vi "Dashboard_Main_Fixed_1366_768.vi"() -> ()   [LabVIEW 2023]
uses:
  <vilib>/event_ctls.llb/eventvkey.ctl
  <vilib>/Rock Robotics/Network Tables/NT Read Numeric Array.vi
  <vilib>/Rock Robotics/WPI/Dashboard/WPI_DashboardLogging Global.vi
panel:
  in  "Camera Settings Right":T1={"Frame Rate"=30, "Compression"=30, "Size"=1, "DB Camera Config"=FALSE} {"Frame Rate" scale=1.0..30.0; "Compression" scale=100.0..-1.0; "Size" items=["640x480", "320x240", "160x120"]}
  in  "Camera Name Right":string(combo)="No Camera Selection"
  out "Camera Perf":string
  in  "Camera Settings":T1={"Frame Rate"=30, "Compression"=30, "Size"=1, "DB Camera Config"=FALSE} {"Frame Rate" scale=1.0..30.0; "Compression" scale=100.0..-1.0; "Size" items=["640x480", "320x240", "160x120"]}
  in  "TCP":refnum<k5>
  in  "Rec Mode":enum32{"Stop", "Record", "Playback"}(radio)
  out "Robot IP":string
  out "Image Message":string="Timeout in Camera Communications"
  in  "Dashboard Tab":T2(tab)
  in  "Select Auto":string(combo)="Select Autonomous ..."
  out "NT Connection":bool
  out "MotorChart R":cluster{"Numeric":dbl, "Numeric":dbl}(graph)
  out "MotorChart L":cluster{"Numeric":dbl, "Numeric":dbl}(graph)
  out "MotorSliders R":cluster{"MotorSlide1":dbl, "MotorSlide2":dbl} {"MotorSlide2" scale=-1.0..1.0 scale format="%#_2e"; "MotorSlide1" scale=-1.0..1.0 scale format="%#_2e"}
  out "MotorSliders L":cluster{"MotorSlide1":dbl, "MotorSlide2":dbl} {"MotorSlide2" scale=-1.0..1.0 scale format="%#_2e"; "MotorSlide1" scale=-1.0..1.0 scale format="%#_2e"}
  out "Gyro":dbl(knob) scale=0.0..360.0
  out "JS1 Z":dbl(slide) scale=-1.0..1.0 scale format="%#_2e"
  out "JS1 Graph":cluster{"X":dbl, "Y":dbl}[](graph)
  out "JS1 Buttons":T3
  out "JS2 Z":dbl(slide) scale=-1.0..1.0 scale format="%#_2e"
  out "JS2 Graph":cluster{"X":dbl, "Y":dbl}[](graph)
  out "JS2 Buttons":T3
  out "Mode":T4(ring)=enum."Auto Disabled"
  out "Right Camera Perf":cluster{"Bandwidth (Mbps)":dbl, "FPS":dbl}
  out "Camera Image Right":T5(plugin-control)
  in  "DB/String 9":string
  in  "DB/String 8":string
  in  "DB/String 7":string
  in  "DB/String 6":string
  in  "DB/String 5":string
  in  "DB/String 4":string
  in  "DB/String 3":string
  in  "DB/String 2":string
  in  "DB/String 1":string
  in  "DB/String 0":string
  in  "DB/Slider 0":dbl(slide) scale=0.0..5.0
  in  "DB/Slider 1":dbl(slide) scale=0.0..5.0
  in  "DB/Slider 2":dbl(slide) scale=0.0..5.0
  in  "DB/Slider 3":dbl(slide) scale=0.0..5.0
  out "DB/LED 3":bool
  out "DB/LED 2":bool
  out "DB/LED 1":bool
  out "DB/LED 0":bool
  in  "DB/Button 3":bool
  in  "DB/Button 2":bool
  in  "DB/Button 1":bool
  in  "DB/Button 0":bool caption="New Name"
  in  "Test Slider":dbl(slide) scale=0.0..100.0 scale format="%#_3g"
  in  "On/Off":bool caption="Solenoid"
  in  "Test Name":u16(ring) items=["Select the test to run..."]
  in  "Test Tree":string(tree)
  in  "Motor":cluster{"Value":dbl, "Enable":bool} {"Value" scale=-1.0..1.0 scale format="%#_3g"}
  out "Progress":T6 {"Test Progress" scale=0.0..100.0}
  in  "Rev/Fwd":cluster{"Forward":bool, "Reverse":bool}
  in  "Test Ring":u16(ring) items=["Monochrome", "Color"]
  in  "CheckList":i32(listbox)
  out "Tree":string(tree)
  out "Camera Image":T5(plugin-control)
  out "Background":bool
  in  "Camera Name":string(combo)="No Camera Selection"
  # "HW"
  # "HW"
  # "Joysticks"
  # "Drive Motors"
  # "Front"
  # "Right"
  # "Left"
  # "Back"
  # "This tab is a great place for autonomous settings and robot-specific values.\nPlace controls and indicators inside this tab and match name to\nDashboard Variables on robot. You can also delete this comment."
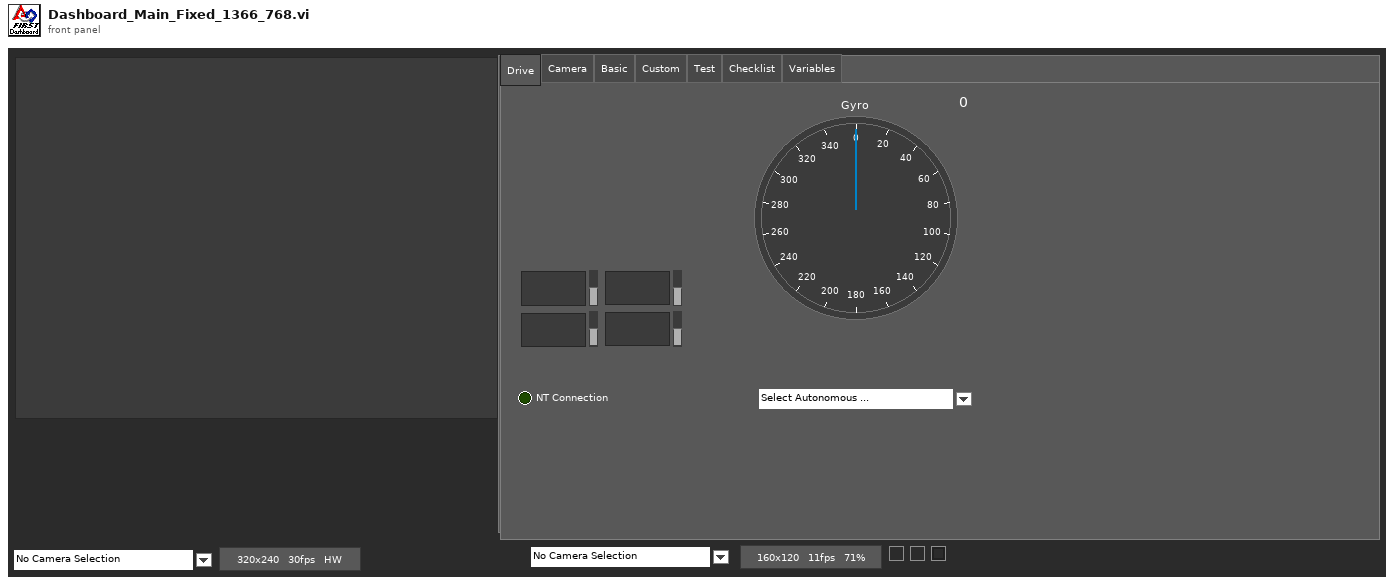
[diagram p1: front panel]
types:
  T1 = cluster{"Frame Rate":i32, "Compression":i32, "Size":u16, "DB Camera Config":bool}
  T2 = enum32{"Drive", "Camera", "Basic", "Custom", "Test", "Checklist", "Variables"}
  T3 = cluster{bool, bool, bool, bool, bool, bool, bool, bool, bool, bool, bool, bool}
  T4 = enum8{"Tele-Op Disabled", "Tele-Op Enabled", "Auto Disabled", "Auto Enabled", "Test Disabled", "Test Enabled", "Disconnected", "No Code", "E-Stop"}
  T5 = typedef "IMAQ Image.ctl" = refnum<image>
  T6 = cluster{"Test Progress":u8, "Test Progress Text":string}
  T7 = cluster{"Save Path":path, "Interval (s)":dbl, "Keep":i32}
  T8 = enum32{"Drive", "Camera", "Basic", "Custom", "Test", "Commands", "Checklist", "Variables"}
  T9 = typedef "Image Type" = u32
  T10 = cluster{"Error Strings":string, "Disable Counts":cluster{u16, u16}, "Rail Faults":cluster{u16, u16, u16}, "Robot IP":string, "DB Mode":u8, "Event Info":cluster{"Name":string, "Type":u8, "Number":u16, "Replay":u8}}
  T11 = cluster{"Storage":cluster{"Disk Free":u64, "RAM Block":u32, "RAM free":u32}, "CPU Utilization":cluster{"CPU % ISR":sgl, "CPU % Time Crit":sgl, "CPU % Timed Str":sgl, "CPU % High":sgl, "CPU % Above":sgl, "CPU % Normal":sgl, "CPU % Low":sgl}, "CAN":cluster{"% Bus Utilization":sgl, "Bus Off Cnt":u32, "TX_FIFO Full Cnt":u32, "Receive Error Cnt":u8, "Transmit Error Cnt":u8}, "HID":cluster{"HID Outputs":u32, "Rumble Low":u16, "Rumble High":u16}[]}
  T12 = cluster{"Status bits":cluster{"Test Mode":bool, "Autonomous":bool, "Enabled":bool, "Code Start":bool, "Brownout":bool, "Reserved 2":bool, "Reserved 3":bool, "E-Stop":bool}, "Code Trace":cluster{"Disabled":bool, "TeleOp":bool, "Auto":bool, "Test":bool}, "Controller Type":enum16{"unknown", "cRIO", "roboRio"}, "Code?":enum16{"unknown", "noCode", "code"}, "Battery V":dbl}
  T13 = cluster{"Control Bits":cluster{"TestMode":bool, "Autonomous":bool, "Enabled":bool, "FMS Present":bool, bool, bool, bool, "E-Stop":bool}, "Team Station ":u8, "Countdown":sgl, "Joystick Values":cluster{"Axes":dbl[], "Buttons":bool[], "POVs":i16[]}[]}
  T14 = cluster{"Axes":dbl[], "Buttons":bool[], "POVs":i16[]}[]
  T15 = cluster{"Axes":dbl[], "Buttons":bool[], "POVs":i16[]}
  T16 = cluster{"Buttons[0]":bool, "Buttons[1]":bool, "Buttons[2]":bool, "Buttons[3]":bool, "Buttons[4]":bool, "Buttons[5]":bool, "Buttons[6]":bool, "Buttons[7]":bool, "Buttons[8]":bool, "Buttons[9]":bool, "Buttons[10]":bool, "Buttons[11]":bool}
  T17 = cluster{"Camera Image":refnum<vi>, "Dashboard Tab":refnum<vi>, "Background":refnum<vi>, "Rec Mode":refnum<vi>, "Test Slider":refnum<vi>, "On/Off ":refnum<vi>, "Test Ring":refnum<vi>, "Rev/Fwd":refnum<vi>, "Test Name":refnum<vi>, "Motor":refnum<vi>, "Progress":refnum<vi>, "CheckList":refnum<vi>, "Tree":refnum<vi>, "Test Tree":refnum<vi>, "Camera Settings":refnum<vi>, "Camera Name":refnum<vi>, "Camera Perf":refnum<vi>, "Camera Settings Right":refnum<vi>, "Camera Name Right":refnum<vi>, "Camera Image Right":refnum<vi>}
  T18 = cluster{"Global Rectangle":i32[], "Contours":cluster{"Contour Type":u32, "ROI Type":u32, "Points":i32[]}[]}
  T19 = cluster{"Camera Name":string, string, "Saved DB Images Info":cluster{"Save Path":path, "Interval (s)":dbl, "Keep":i32}}
  T20 = cluster{"Camera Name Right":string, string, "Saved DB Images Info":cluster{"Save Path":path, "Interval (s)":dbl, "Keep":i32}}
  T21 = cluster{"Operation":enum16{"Update", "Clear"}, "Color Box":u32}[]
  T22 = typedef "eventvkey.ctl" = enum16{"ASCII", "Enter", "Return", "Shift", "Ctrl", "Alt", "Cmd", "Opt", "Caps", "NumLock", "Clear", "Break", "Up", "Down", "Left", "Right", "Insert", "Delete", "Home", "End", "PageUp", "PageDown", "Escape", "Help", "Pause", "ScrollLock", "F1", "F2", "F3", "F4", "F5", "F6", "F7", "F8", "F9", "F10", "F11", "F12", "F13", "F14", "F15", "F16", "F17", "F18", "F19", "F20", "F21", "F22", "F23", "F24", "Play", "VolumeUp", "VolumeDown", "Mute", "Two Byte Char"}
  T23 = cluster{"Image Size":bool, "Image Type":bool, "Pixel Value":bool, "ROI Information":bool, "Zoom Factor":bool}
  T24 = cluster{"Operation":enum16{"Update", "Clear"}, "Color Box":u32}
  T25 = cluster{"Shift":bool, "Ctrl":bool, "Alt":bool, "Cmd":bool, "Opt":bool}
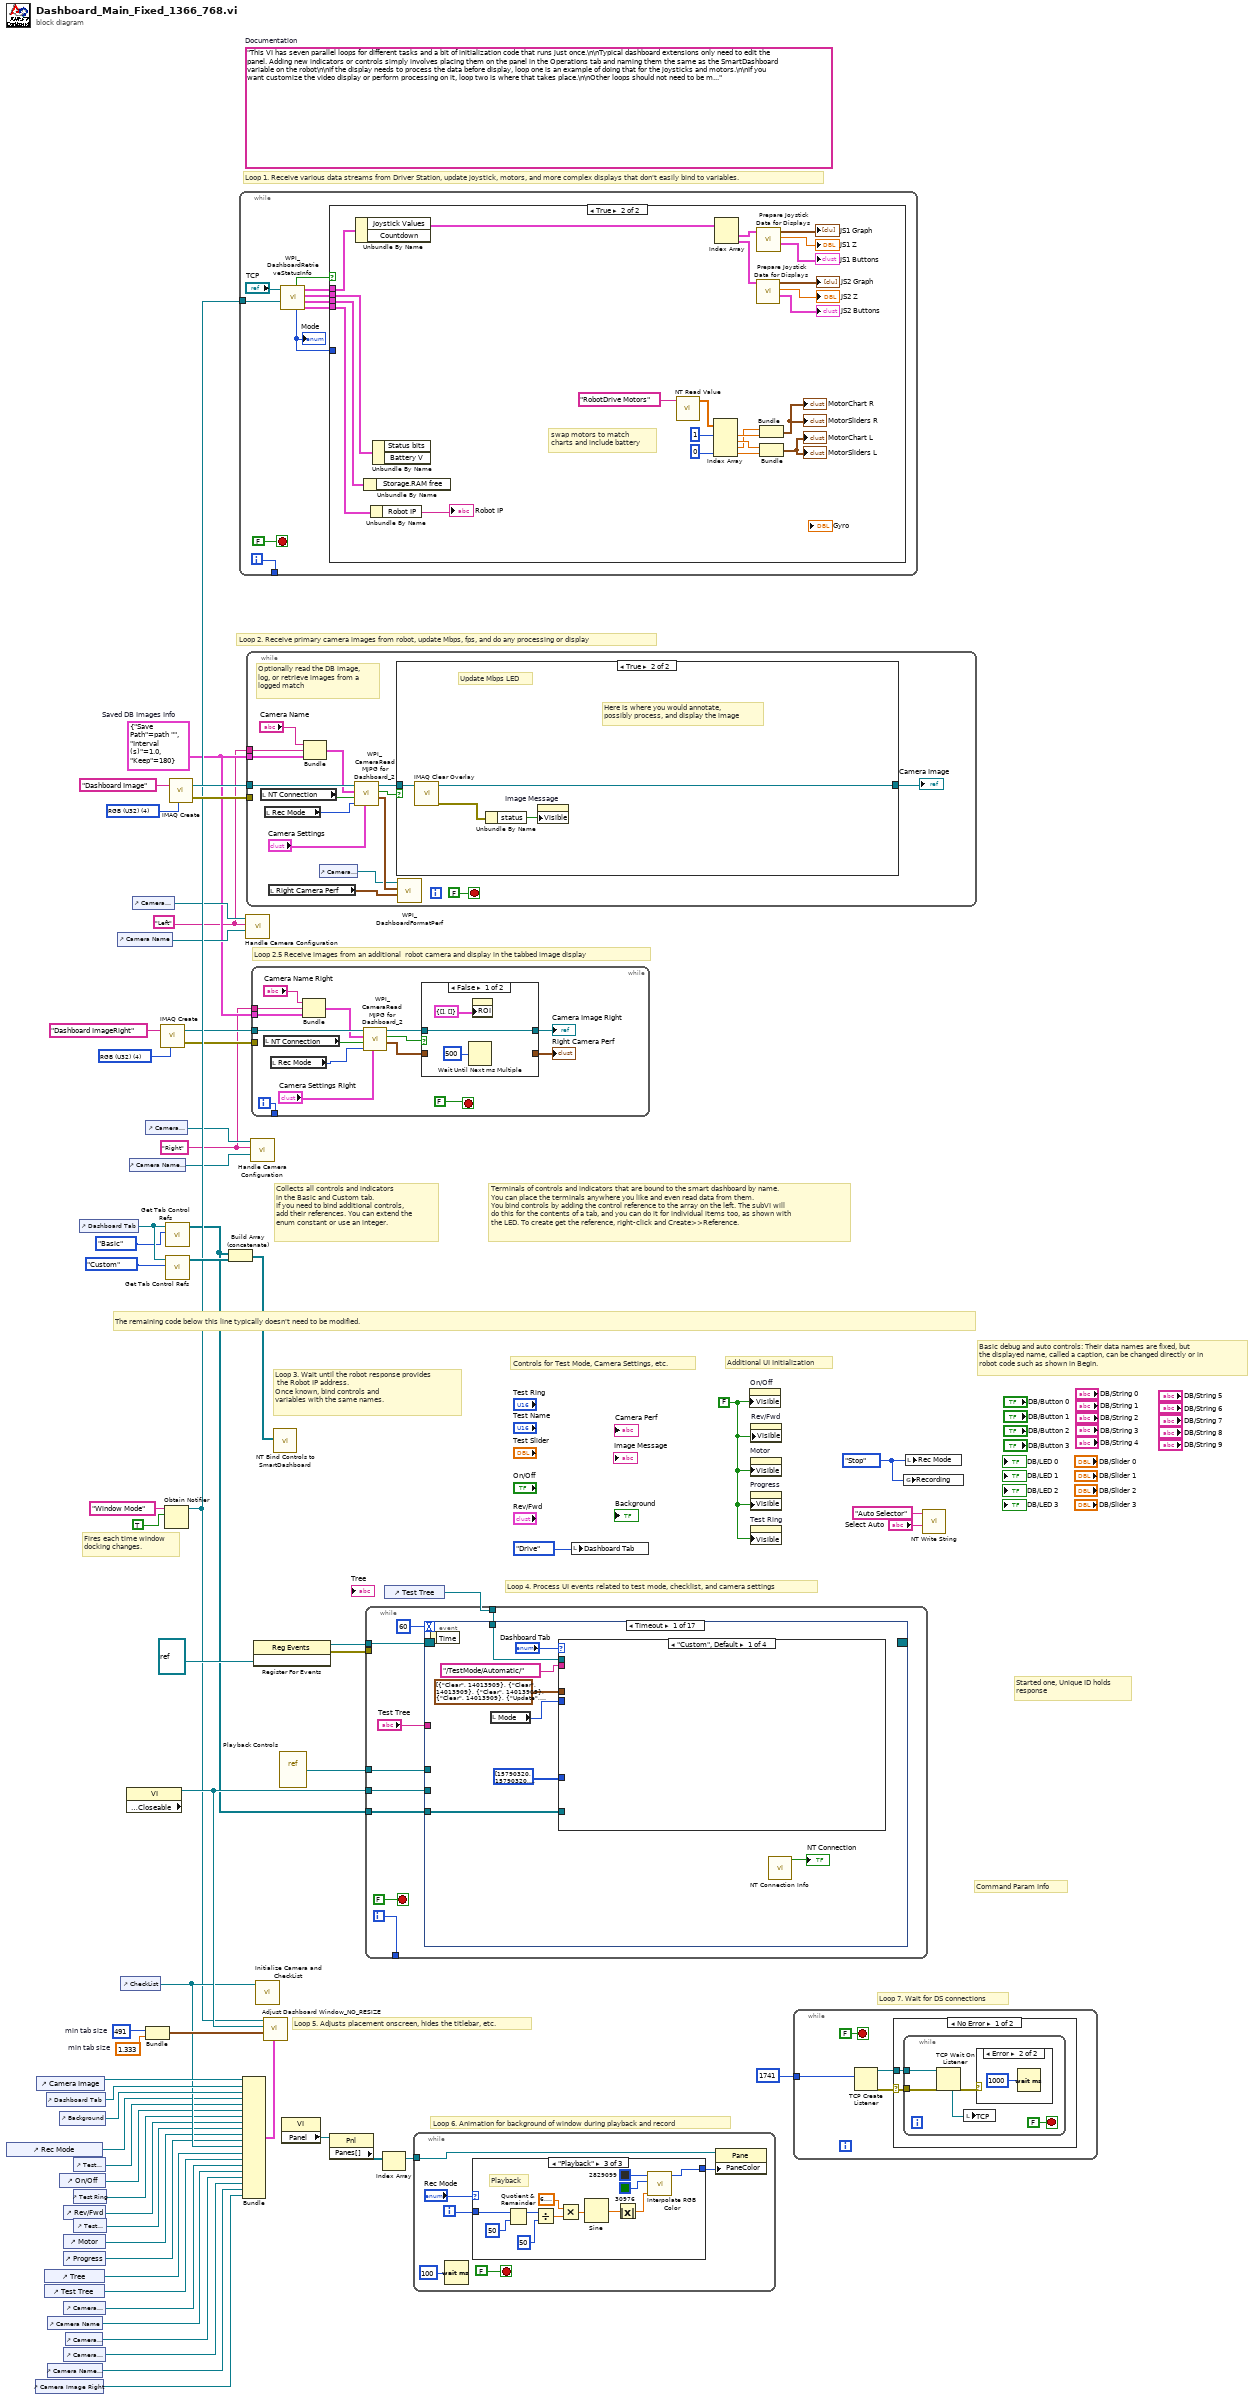
[diagram p0: block diagram]
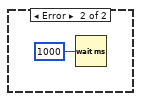
[diagram p4: hidden frame]
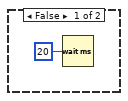
[diagram p5: hidden frame]
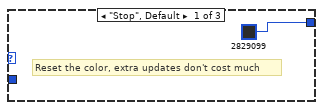
[diagram p6: hidden frame]
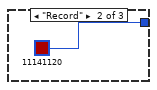
[diagram p7: hidden frame]
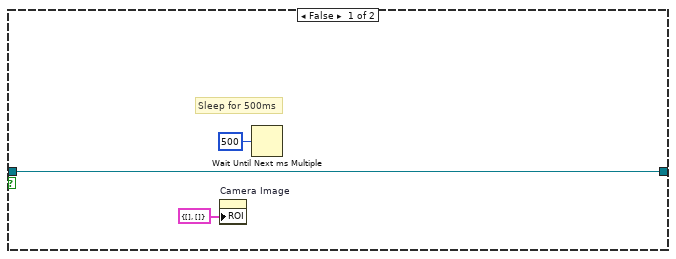
[diagram p8: hidden frame]
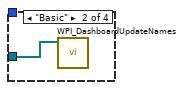
[diagram p9: hidden frame]
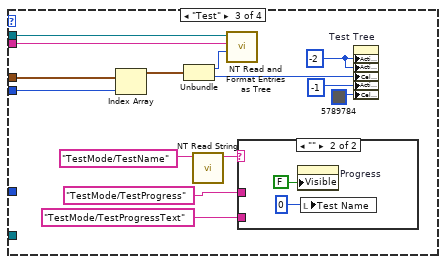
[diagram p10: hidden frame]
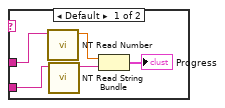
[diagram p11: hidden frame]
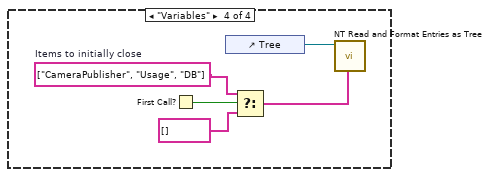
[diagram p12: hidden frame]
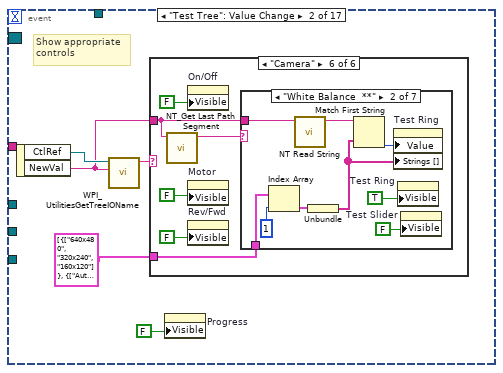
[diagram p13: hidden frame]
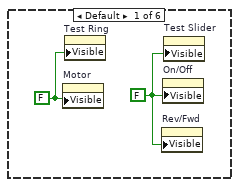
[diagram p14: hidden frame]
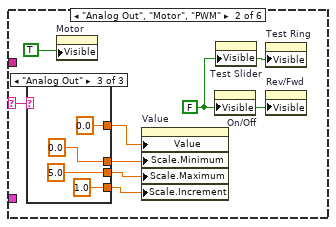
[diagram p15: hidden frame]
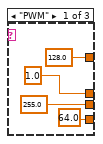
[diagram p16: hidden frame]
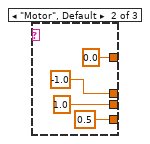
[diagram p17: hidden frame]
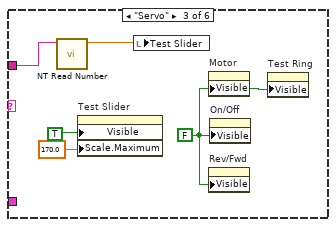
[diagram p18: hidden frame]
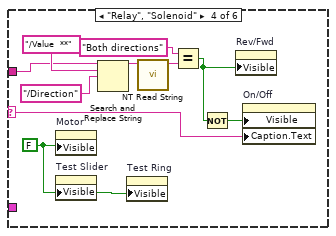
[diagram p19: hidden frame]
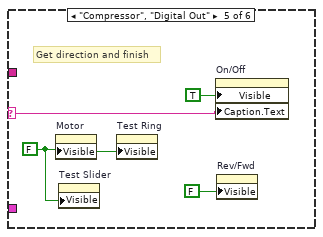
[diagram p20: hidden frame]
diagram:
  w3 = T7 {"Save Path"=path "", "Interval (s)"=1.0, "Keep"=180}  # Saved DB Images Info
  w2 = "Right"
  w1 = "Left"
  w13 = T9 4 items=["Grayscale (U8)", "Grayscale (I16)", "Grayscale (SGL)", "Complex (CSG)", "RGB (U32)", "HSL (U32)", "RGB (U64)"] ("Image Type")
  w42 = 491  # min tab size
  w41 = 1.333  # min tab size
  w49 = enum32{"Stop", "Record", "Playback"}."Stop" ("Rec Mode")
  w26 = FALSE ("Visible")
  (unwired) "This VI has seven parallel loops for different tasks and a bit of initialization code that runs just once.\n\nTypical dashboard extensions only need to edit the panel. Adding new indicators or controls simply involves placing them on the panel in the Operations tab and naming them the same as the SmartDashboard variable on the robot\n\nIf the display needs to process the data before display, loop one is an example of doing that for the joysticks and motors.\n\nIf you want customize the video display or perform processing on it, loop two is where that takes place.\n\nOther loops should not need to be modified. They are pretty standard, and document the task they perform."  # Documentation
  w63 = T9 4 items=["Grayscale (U8)", "Grayscale (I16)", "Grayscale (SGL)", "Complex (CSG)", "RGB (U32)", "HSL (U32)", "RGB (U64)"] ("Image Type")
  # "Loop 2.5 Receive images from an additional  robot camera and display in the tabbed image display"
  # "Command Param Info"
  # "Started one, Unique ID holds\nresponse"
  # "Loop 7. Wait for DS connections"
  # "Basic debug and auto controls: Their data names are fixed, but\nthe displayed name, called a caption, can be changed directly or in\nrobot code such as shown in Begin."
  # "Controls for Test Mode, Camera Settings, etc."
  # "Additional UI Initialization"
  # "Loop 6. Animation for background of window during playback and record"
  # "Fires each time window\ndocking changes."
  # "Collects all controls and indicators\nin the Basic and Custom tab.\nIf you need to bind additional controls,\nadd their references. You can extend the\nenum constant or use an integer."
  # "The remaining code below this line typically doesn't need to be modified."
  # "Loop 4. Process UI events related to test mode, checklist, and camera settings"
  # "Terminals of controls and indicators that are bound to the smart dashboard by name.\nYou can place the terminals anywhere you like and even read data from them.\nYou bind controls by adding the control reference to the array on the left. The subVI will\ndo this for the contents of a tab, and you can do it for individual items too, as shown with\nthe LED. To create get the reference, right-click and Create>>Reference."
  # "Loop 3. Wait until the robot response provides\n the Robot IP address.\nOnce known, bind controls and\nvariables with the same names."
  # "Loop 5. Adjusts placement onscreen, hides the titlebar, etc."
  # "Loop 1. Receive various data streams from Driver Station, update joystick, motors, and more complex displays that don't easily bind to variables."
  # "Loop 2. Receive primary camera images from robot, update Mbps, fps, and do any processing or display"
  n1 = control-ref of="Rec Mode"() -> (w32:refnum<vi>)
  n2 = control-ref of="Camera Image Right"() -> (w6:refnum<vi>)
  n3 = control-ref of="Camera Image"() -> (w44:refnum<vi>)
  n4 = control-ref of="Tree"() -> (w36:refnum<vi>)
  n5 = control-ref of="Test Tree"() -> (w35:refnum<vi>)
  n6 = control-ref of="Dashboard Tab"() -> (w43:refnum<vi>)
  n7 = control-ref of="Camera Name"() -> (w19:refnum<vi>)
  n8 = control-ref of="Camera Name Right"() -> (w7:refnum<vi>)
  n9 = control-ref of="Background"() -> (w39:refnum<vi>)
  n10 = control-ref of="On/Off"() -> (w30:refnum<vi>)
  n11 = control-ref of="Progress"() -> (w27:refnum<vi>)
  n12 = control-ref of="Camera Settings"() -> (w20:refnum<vi>)
  n13 = control-ref of="Camera Settings Right"() -> (w8:refnum<vi>)
  n14 = control-ref of="Rev/Fwd"() -> (w28:refnum<vi>)
  n15 = control-ref of="Motor"() -> (w33:refnum<vi>)
  n16 = control-ref of="Camera Perf"() -> (w18:refnum<vi>)
  n17 = control-ref of="Test Slider"() -> (w31:refnum<vi>)
  n18 = control-ref of="Test Ring"() -> (w29:refnum<vi>)
  n19 = control-ref of="Test Name"() -> (w34:refnum<vi>)
  n20 = control-ref of="Dashboard Tab"() -> (w47:refnum<vi>)
  n21 = control-ref of="Camera Name"() -> (w21:refnum<vi>)
  n22 = control-ref of="CheckList"() -> (w37:refnum<vi>)
  n23 = property class="VI" props=["Front Panel.Closeable"]() -> (reference out=w48:refnum<vi>)  [unwired: 2 in, 2 out]
  n24 = control-ref of="Camera Name Right"() -> (w9:refnum<vi>)
  n25 = control-ref of="Camera Settings"() -> (w22:refnum<vi>)
  n26 = control-ref of="Camera Settings Right"() -> (w10:refnum<vi>)
  n27 = Bundle("min tab size"=w42, "min tab size"=w41) -> (w40:cluster{"min tab size":i32, "min tab size":dbl})  [unwired: 1 in]
  n28 = call "IMAQ Create"("Image Name"="Dashboard ImageRight", "Image Type"=w13) -> ("New Image"=w12:T5, "error out"=w11:errorcluster)  [unwired: 2 in, 1 out]
  n29 = Obtain Notifier(name (unnamed)="Window Mode", notification data type=TRUE) -> (notifier out=w25:refnum<notifier>)  [unwired: 2 in, 2 out]
  n30 = call <vilib>:"Get Tab Control Refs.vi"("Page Index"=T8."Basic" ("Dashboard Tab"), "TabControl in"=w47) -> ("ControlsOnPage"=w17:refnum<vi>[])  [unwired: 9 in]
  n31 = call <vilib>:"Get Tab Control Refs.vi"("Page Index"=T8."Custom" ("Dashboard Tab"), "TabControl in"=w47) -> ("ControlsOnPage"=w46:refnum<vi>[])  [unwired: 9 in]
  n32 = call "IMAQ Create"("Image Name"="Dashboard Image", "Image Type"=w63) -> ("New Image"=w61:T5, "error out"=w60:errorcluster)  [unwired: 2 in, 1 out]
  n33 = Build Array (concatenate)(w17, w46) -> (w45:refnum<vi>[])
  n34 = while {
    tunnel: [w72] -> _
    tunnel: w25 -> [w64]
    i -> [w72]
    stop <- FALSE stop-if-true
    n35 = call <vilib>:"WPI_DashboardRetrieveStatusInfo.vi"("Window Mode Notifier"=w64, "TCP Cnx"="TCP") -> ("Power and Errors"=w67:T10, "Robot Metrics"=w70:T11, "Status Info"=w71:T12, "Control Info"=w68:T13, "Robot Mode"=w66:T4, "Process?"=w69:bool)  [unwired: 4 in]
    "Mode" <- w66
    n36 = case shown="True" w69 {
      tunnel: w71 -> [_ w98]
      tunnel: w70 -> [_ w97]
      tunnel: w68 -> [_ w96]
      tunnel: w67 -> [_ w95]
      tunnel: w66 -> [_ _]
      frame False {
        n37 = Wait (ms)(milliseconds to wait=u32 20) -> ()  [unwired: 1 out]
      }
      frame True {
        # "swap motors to match\ncharts and include battery"
        n38 = Unbundle By Name(w96) -> ("Joystick Values"=w86:T14)  [unwired: 1 out]
        n39 = Unbundle By Name(w97) -> ()  [unwired: 1 out]
        n40 = Unbundle By Name(w95) -> ("Robot IP"=→"Robot IP":string)
        n41 = Unbundle By Name(w98) -> ()  [unwired: 2 out]
        n42 = call-poly <vilib>:"NT Read Value.vi"("name"="RobotDrive Motors" ("Name")) -> ("value"=w76:dbl[])  [unwired: 8 in, 2 out]
        n43 = Index Array(array=w76, index #1=1, index #4=0) -> (element #1=w90:dbl, element #2=w91:dbl, element #3=w89:dbl, element #4=w94:dbl)  [unwired: 2 in]
        n44 = Index Array(array=w86) -> (element #1=w85:T15, element #2=w81:T15)  [unwired: 2 in]
        n45 = call "Prepare Joystick Data for Displays.vi"("Joystick Values"=w81) -> ("Buttons"=→"JS2 Buttons":T16, "Z Axis"=→"JS2 Z":dbl, "Cartesian Data"=→"JS2 Graph":cluster{"X axis":dbl, "X axis":dbl}[])  [unwired: 8 in]
        n46 = call "Prepare Joystick Data for Displays.vi"("Joystick Values"=w85) -> ("Buttons"=→"JS1 Buttons":T16, "Z Axis"=→"JS1 Z":dbl, "Cartesian Data"=→"JS1 Graph":cluster{"X axis":dbl, "X axis":dbl}[])  [unwired: 8 in]
        n47 = Bundle("Numeric"=w89, "Numeric"=w90) -> (→"MotorChart R" →"MotorSliders R":cluster{"Numeric":dbl, "Numeric":dbl})  [unwired: 1 in]
        n48 = Bundle("Numeric"=w91, "Numeric"=w94) -> (→"MotorChart L" →"MotorSliders L":cluster{"Numeric":dbl, "Numeric":dbl})  [unwired: 1 in]
      }
    }
  }
  n49 = Bundle("Camera Image"=w44, "Dashboard Tab"=w43, "Background"=w39, "Rec Mode"=w32, "Test Slider"=w31, "On/Off"=w30, "Test Ring"=w29, "Rev/Fwd"=w28, "Test Name"=w34, "Motor"=w33, "Progress"=w27, "CheckList"=w37, "Tree"=w36, "Test Tree"=w35, "Camera Settings"=w20, "Camera Name"=w19, "Camera Perf"=w18, "Camera Settings Right"=w8, "Camera Name Right"=w7, "Camera Image Right"=w6) -> (w38:T17)  [unwired: 1 in]
  n50 = call "Handle Camera Configuration.vi"("CameraNameRef"=w21, "Display Name"=w1, "ClusterRef"=w22) -> ()  [unwired: 9 in]
  n51 = while {
    tunnel: w61 -> [w112]
    tunnel: w60 -> [_]
    tunnel: w3 -> [w105]
    tunnel: w1 -> [w102]
    stop <- FALSE stop-if-true
    # "Optionally read the DB image,\nlog, or retrieve images from a\nlogged match"
    n52 = local read "NT Connection"() -> (w106:bool)
    n53 = local read "Rec Mode"() -> (w109:enum32{"Stop", "Record", "Playback"})
    n54 = local read "Right Camera Perf"() -> (w100:cluster{"Bandwidth (Mbps)":dbl, "FPS":dbl})
    n55 = Bundle("Camera Name"="Camera Name", w102, "Saved DB Images Info"=w105) -> (w104:T19)  [unwired: 1 in]
    n56 = control-ref of="Camera Perf"() -> (w99:refnum<vi>)
    n57 = call <vilib>:"WPI_CameraRead MJPG for Dashboard_2.vi"("Camera Settings"="Camera Settings", "Rec Mode"=w109, "NT Connection"=w106, "Capture Info"=w104, "Image in"=w112) -> ("perf info"=w101:cluster{"Bandwidth (Mbps)":dbl, "fps":dbl}, "Active"=w110:bool, "Image\\ out"=w111:T5)  [unwired: 4 in]
    n58 = case shown="True" w110 {
      tunnel: w111 -> [w115 w118]
      tunnel: [w115 w117] -> w107
      frame False {
        # "Sleep for 500ms"
        n59 = property on="Camera Image" class="ImageControl"("ROI"=T18 {"Global Rectangle"=[], "Contours"=[]}) -> ()  [unwired: 2 in, 2 out]
        n60 = Wait Until Next ms Multiple(millisecond multiple=u32 500) -> ()  [unwired: 1 out]
      }
      frame True {
        # "Here is where you would annotate,\npossibly process, and display the image"
        # "Update Mbps LED"
        n61 = call "IMAQ Clear Overlay"("Image"=w118) -> ("error out"=w119:errorcluster, "Image Out"=w117:T5)  [unwired: 2 in, 7 out]
        n62 = Unbundle By Name(w119) -> ("status"=w120:bool)
        n63 = property on="Image Message" class="Str"("Visible"=w120) -> ()  [unwired: 2 in, 2 out]
      }
    }
    "Camera Image" <- w107
    n64 = call <vilib>:"WPI_DashboardFormatPerf.vi"("Right Camera Perf"=w100, "Performance"=w101, "String in"=w99) -> ()  [unwired: 9 in]
  }
  n65 = call "Handle Camera Configuration.vi"("CameraNameRef"=w9, "Display Name"=w2, "ClusterRef"=w10) -> ()  [unwired: 9 in]
  n66 = while {
    tunnel: w12 -> [w135]
    tunnel: w11 -> [_]
    tunnel: [w130] -> _
    tunnel: w3 -> [w126]
    tunnel: w2 -> [w123]
    i -> [w130]
    stop <- FALSE stop-if-true
    n67 = local read "NT Connection"() -> (w127:bool)
    n68 = local read "Rec Mode"() -> (w134:enum32{"Stop", "Record", "Playback"})
    n69 = Bundle("Camera Name Right"="Camera Name Right", w123, "Saved DB Images Info"=w126) -> (w125:T20)  [unwired: 1 in]
    n70 = call <vilib>:"WPI_CameraRead MJPG for Dashboard_2.vi"("Camera Settings"="Camera Settings Right", "Rec Mode"=w134, "NT Connection"=w127, "Capture Info"=w125, "Image in"=w135) -> ("perf info"=w121:cluster{"Bandwidth (Mbps)":dbl, "fps":dbl}, "Active"=w129:bool, "Image\\ out"=w132:T5)  [unwired: 4 in]
    n71 = case shown="False" w129 {
      tunnel: w132 -> [w137 w140]
      tunnel: [w137 w140] -> w128
      tunnel: [_ w139] -> w122
      tunnel: w121 -> [_ w139]
      frame False {
        n72 = Wait Until Next ms Multiple(millisecond multiple=u32 500) -> ()  [unwired: 1 out]
        n73 = property on="Camera Image Right" class="ImageControl"("ROI"=T18 {"Global Rectangle"=[], "Contours"=[]}) -> ()  [unwired: 2 in, 2 out]
      }
      frame True {
      }
    }
    "Camera Image Right" <- w128
    "Right Camera Perf" <- w122
  }
  n74 = register-events(refnum<vi> refnum) -> (reference out=w52:refnum<event-registration>, error out=w51:errorcluster)  [unwired: 2 in]
  n75 = call "Initialize Camera and CheckList.vi"("ListBox in"=w37) -> ()  [unwired: 11 in]
  n76 = call "Adjust Dashboard Window_NO_RESIZE.vi"("Sizing Refnums"=w38, "Size Constraints"=w40, "VI"=w48, "WIn Mode"=w25) -> ()  [unwired: 8 in]
  n77 = call <vilib>:"NT Bind Controls to SmartDashboard.vi"("Bound Control Refs"=w45) -> ()  [unwired: 11 in]
  n78 = vi-ref "Playback Controls.vi"() -> (w53:refnum<vi>)
  n79 = property class="VI"() -> ("Panel"=w55:refnum<vi>)  [unwired: 2 in, 2 out]
  n80 = property class="Pnl"(reference=w55) -> ("Panes[]"=w56:refnum<vi>[])  [unwired: 1 in, 2 out]
  n81 = Index Array(array=w56) -> (element=w54:refnum<vi>)  [unwired: 1 in]
  n82 = control-ref of="Test Tree"() -> (w57:refnum<vi>)
  n83 = while {
    tunnel: [w146] -> _
    tunnel: w57 -> [w145]
    tunnel: w53 -> [w144]
    tunnel: w52 -> [w143]
    tunnel: w51 -> [_]
    tunnel: w48 -> [w142]
    tunnel: w17 -> [w141]
    i -> [w146]
    stop <- FALSE stop-if-true
    n84 = event shown="[0] Timeout" {
      selector: w143 -> [_ _ _ _ _ _ _ _ _ _ _ _ _ _ _ _ _]
      dyn-events: [_ _ _ _ _ _ _ _ _ _ _ _ _ w351 _ _ _] -> _
      timeout: u32 60 ("milliseconds to wait") -> [_ _ _ _ _ _ _ _ _ _ _ _ _ _ _ _ _]
      tunnel: w145 -> [w156 _ _ _ _ _ _ _ _ _ _ _ _ _ _ _ _]
      tunnel: "Test Tree" -> [_ _ _ _ _ _ _ _ w324 w331 w332 w335 w342 _ _ _ _]
      tunnel: w144 -> [_ _ _ _ _ _ _ _ _ _ _ _ _ w353 _ w368 _]
      tunnel: w142 -> [_ _ _ _ _ _ _ _ _ _ _ _ _ w349 _ _ _]
      tunnel: w141 -> [w151 _ _ _ _ _ _ _ _ _ _ _ _ _ _ _ _]
      event Timeout {
        n85 = event-data() -> ()  [unwired: 1 in, 1 out]
        n86 = local read "Mode"() -> (w154:T4)
        n87 = case shown="\"Custom\", Default" "Dashboard Tab" {
          tunnel: w156 -> [_ _ w172 _]
          tunnel: "/TestMode/Automatic/" ("Name Pattern") -> [_ _ w171 _]
          tunnel: T21 [{"Operation"=enum."Clear", "Color Box"=14013909}, {"Operation"=enum."Clear", "Color Box"=14013909}, {"Operation"=enum."Clear", "Color Box"=14013909}, {"Operation"=enum."Clear", "Color Box"=14013909}, {"Operation"=enum."Update", "Color Box"=14013909}, {"Operation"=enum."Update", "Color Box"=16777215}, {"Operation"=enum."Clear", "Color Box"=14013909}, {"Operation"=enum."Clear", "Color Box"=14013909}, {"Operation"=enum."Clear", "Color Box"=14013909}] -> [_ _ w164 _]
          tunnel: w154 -> [_ _ w163 _]
          tunnel: u32[] [15790320, 15790320, 15790320, 15790320, 16777215, 16777215, 15790320, 15790320, 15790320] -> [_ _ _ _]
          tunnel: w151 -> [_ w158 _ _]
          frame "Custom", Default {
          }
          frame "Basic" {
            n88 = call <vilib>:"WPI_DashboardUpdateNames.vi"("Controls on Tab"=w158) -> ()  [unwired: 11 in]
          }
          frame "Test" {
            w170 = -2 ("Active Item:Row Number")
            n89 = Index Array(array=w164, index=w163) -> (element=w165:T24)
            n90 = Unbundle(w165) -> ("Operation"=w166:enum16{"Update", "Clear"}, "Color Box"=w167:u32)
            n91 = call <vilib>:"NT Read String.vi"("name"="TestMode/TestName" ("Name")) -> ("value"=w161:string)  [unwired: 8 in, 2 out]
            n92 = call <vilib>:"NT Read and Format Entries as Tree.vi"("Operation"=w166, "Name Pattern"=w171, "Tree Refnum"=w172) -> ()  [unwired: 7 in, 2 out]
            n93 = case shown="\"\"" w161 {
              tunnel: "TestMode/TestProgress" ("Name") -> [w174 _]
              tunnel: "TestMode/TestProgressText" ("Name") -> [w173 _]
              frame Default {
                n94 = call <vilib>:"NT Read Number.vi"("name"=w174) -> ("value"=w175:dbl)  [unwired: 8 in, 2 out]
                n95 = call <vilib>:"NT Read String.vi"("name"=w173) -> ("value"=w176:string)  [unwired: 8 in, 2 out]
                n96 = Bundle("value"=w175, "value"=w176) -> (→"Progress":cluster{"value":dbl, "value":string})  [unwired: 1 in]
              }
              frame "" {
                n97 = property on="Progress" class="Clust (strict)"("Visible"=FALSE) -> ()  [unwired: 2 in, 2 out]
                n98 = local write "Test Name"(u16 0) -> ()
              }
            }
            n99 = property on="Test Tree" class="Tree (strict)"("Active Item Row Number"=w170, "ActiveColNum"=w170, "CellBG"=w167, "Active Item Row Number"=-1 ("Active Item:Row Number"), "CellBG"=u32 5789784 ("Color Box")) -> ()  [unwired: 2 in, 2 out]
          }
          frame "Variables" {
            w182 = string[] ["CameraPublisher", "Usage", "DB"]  # Items to initially close
            n100 = First Call?() -> (First Call?: T/F=w183:bool)
            n101 = control-ref of="Tree"() -> (w184:refnum<vi>)
            n102 = Select(t=w182, s=w183, f=string[] []) -> (s? t:f=w180:string[])
            n103 = call <vilib>:"NT Read and Format Entries as Tree.vi"("Tags to  Close"=w180, "Tree Refnum"=w184) -> ()  [unwired: 8 in, 2 out]
          }
        }
        n104 = call <vilib>:"NT Connection Info.vi"() -> ("Connected"=→"NT Connection":bool)  [unwired: 11 in]
      }
      event "Test Tree": Value Change {
        # "Show appropriate\ncontrols"
        n105 = event-data() -> ("CtlRef"=w188:refnum<vi>, "NewVal"=w186:string)  [unwired: 1 in]
        n106 = call <vilib>:"WPI_UtilitiesGetTreeIOName.vi"("NewVal"=w186, "TreeControl in"=w188) -> ("I/O Name"=w189:string)  [unwired: 9 in]
        n107 = case shown="\"Camera\"" w189 {
          selector: w189 -> [_ w196 _ w218 w227 _]
          tunnel: w186 -> [_ _ w215 w217 _ w234]
          tunnel: cluster{string[]}[] [{["640x480", "320x240", "160x120"]}, {["Auto", "Fixed indoor", "Fixed outdoor 1", "Fixed outdoor 2", "Fixed fluorescent 1", "Fixed fluorescent 2", "Hold current"]}, {["Auto", "Flicker-free 50 Hz", "Flicker-free 60 Hz", "Hold current"]}, {["None", "Prioritize frame rate", "Prioritize image quality"]}, {["Monochrome", "Color"]}] -> [_ _ _ _ _ w233]
          frame Default {
            w191 = FALSE ("Visible")
            w190 = FALSE ("Visible")
            n108 = property on="Motor" class="Clust (strict)"("Visible"=w190) -> ()  [unwired: 2 in, 2 out]
            n109 = property on="Test Ring" class="Ring (strict)"("Visible"=w190) -> ()  [unwired: 2 in, 2 out]
            n110 = property on="Rev/Fwd" class="Clust (strict)"("Visible"=w191) -> ()  [unwired: 2 in, 2 out]
            n111 = property on="On/Off" class="Bool (strict)"("Visible"=w191) -> ()  [unwired: 2 in, 2 out]
            n112 = property on="Test Slider" class="Slide (strict)"("Visible"=w191) -> ()  [unwired: 2 in, 2 out]
          }
          frame "Analog Out", "Motor", "PWM" {
            w197 = FALSE ("Visible")
            n113 = case shown="\"Analog Out\"" w196 {
              tunnel: [1.0 ("Value") -1.0 ("Value") 0.0 ("Value")] -> w195
              tunnel: [255.0 ("Value") 1.0 ("Value") 5.0 ("Value")] -> w194
              tunnel: [128.0 ("Value") 0.0 ("Value") 0.0 ("Value")] -> w193
              tunnel: [64.0 ("Value") 0.5 ("Value") 1.0 ("Value")] -> w192
              frame "PWM" {
              }
              frame "Motor", Default {
              }
              frame "Analog Out" {
              }
            }
            n114 = property on="Motor" class="Clust (strict)"("Visible"=TRUE) -> ()  [unwired: 2 in, 2 out]
            n115 = property on="Value" class="Slide (strict)"("Value"=w193, "Scale.Minimum"=w195, "Scale.Maximum"=w194, "Scale.Increment"=w192) -> ()  [unwired: 2 in, 2 out]
            n116 = property on="On/Off" class="Bool (strict)"("Visible"=w197) -> ()  [unwired: 2 in, 2 out]
            n117 = property on="Test Slider" class="Slide (strict)"("Visible"=w197) -> ()  [unwired: 2 in, 2 out]
            n118 = property on="Test Ring" class="Ring (strict)"("Visible"=w197) -> ()  [unwired: 2 in, 2 out]
            n119 = property on="Rev/Fwd" class="Clust (strict)"("Visible"=w197) -> ()  [unwired: 2 in, 2 out]
          }
          frame "Servo" {
            w213 = FALSE ("Visible")
            n120 = call <vilib>:"NT Read Number.vi"("name"=w215) -> ("value"=w214:dbl)  [unwired: 8 in, 2 out]
            n121 = property on="Test Slider" class="Slide (strict)"("Visible"=TRUE, "Scale.Maximum"=170.0 ("Scale.Range:Maximum")) -> ()  [unwired: 2 in, 2 out]
            n122 = local write "Test Slider"(w214) -> ()
            n123 = property on="Motor" class="Clust (strict)"("Visible"=w213) -> ()  [unwired: 2 in, 2 out]
            n124 = property on="Rev/Fwd" class="Clust (strict)"("Visible"=w213) -> ()  [unwired: 2 in, 2 out]
            n125 = property on="On/Off" class="Bool (strict)"("Visible"=w213) -> ()  [unwired: 2 in, 2 out]
            n126 = property on="Test Ring" class="Ring (strict)"("Visible"=w213) -> ()  [unwired: 2 in, 2 out]
          }
          frame "Relay", "Solenoid" {
            w216 = FALSE ("Visible")
            n127 = property on="Motor" class="Clust (strict)"("Visible"=w216) -> ()  [unwired: 2 in, 2 out]
            n128 = property on="Test Slider" class="Slide (strict)"("Visible"=w216) -> ()  [unwired: 2 in, 2 out]
            n129 = Search and Replace String(input string=w217, search string="/Value  **", replace string="/Direction") -> (result string=w223:string)  [unwired: 5 in, 3 out]
            n130 = property on="Test Ring" class="Ring (strict)"("Visible"=w216) -> ()  [unwired: 2 in, 2 out]
            n131 = call <vilib>:"NT Read String.vi"("name"=w223) -> ("value"=w221:string)  [unwired: 8 in, 2 out]
            n132 = Equal?(x="Both directions", y=w221) -> (x = y?=w219:bool)
            n133 = Not(x=w219) -> (.not. x?=w220:bool)
            n134 = property on="Rev/Fwd" class="Clust (strict)"("Visible"=w219) -> ()  [unwired: 2 in, 2 out]
            n135 = property on="On/Off" class="Bool (strict)"("Visible"=w220, "Caption.Text"=w218) -> ()  [unwired: 2 in, 2 out]
          }
          frame "Compressor", "Digital Out" {
            w226 = FALSE ("Visible")
            # "Get direction and finish"
            n136 = property on="Motor" class="Clust (strict)"("Visible"=w226) -> ()  [unwired: 2 in, 2 out]
            n137 = property on="Test Slider" class="Slide (strict)"("Visible"=w226) -> ()  [unwired: 2 in, 2 out]
            n138 = property on="Test Ring" class="Ring (strict)"("Visible"=w226) -> ()  [unwired: 2 in, 2 out]
            n139 = property on="On/Off" class="Bool (strict)"("Visible"=TRUE, "Caption.Text"=w227) -> ()  [unwired: 2 in, 2 out]
            n140 = property on="Rev/Fwd" class="Clust (strict)"("Visible"=FALSE) -> ()  [unwired: 2 in, 2 out]
          }
          frame "Camera" {
            n141 = call <vilib>:"NT_Get Last Path Segment.vi"("String in"=w234) -> ("String out"=w235:string)  [unwired: 10 in]
            n142 = property on="On/Off" class="Bool (strict)"("Visible"=FALSE) -> ()  [unwired: 2 in, 2 out]
            n143 = property on="Motor" class="Clust (strict)"("Visible"=FALSE) -> ()  [unwired: 2 in, 2 out]
            n144 = property on="Rev/Fwd" class="Clust (strict)"("Visible"=FALSE) -> ()  [unwired: 2 in, 2 out]
            n145 = case shown="\"White Balance  **\"" w235 {
              tunnel: w234 -> [w241 w250 w259 w268 w277 _ w283]
              tunnel: w233 -> [w239 w247 w256 w265 w274 _ _]
              frame "Size  **" {
                n146 = Index Array(array=w239) -> (element=w238:cluster{string[]})  [unwired: 1 in]
                n147 = call <vilib>:"NT Read String.vi"("name"=w241) -> ("value"=w240:string)  [unwired: 8 in, 2 out]
                n148 = Unbundle(w238) -> (w236:string[])
                n149 = Match First String(2:w236, 3:w240) -> (0:w237:i32)  [unwired: 1 out]
                n150 = property on="Test Ring" class="Ring (strict)"("Value"=w237, "Strings []"=w236) -> ()  [unwired: 2 in, 2 out]
                n151 = property on="Test Ring" class="Ring (strict)"("Visible"=TRUE) -> ()  [unwired: 2 in, 2 out]
                n152 = property on="Test Slider" class="Slide (strict)"("Visible"=FALSE) -> ()  [unwired: 2 in, 2 out]
              }
              frame "White Balance  **" {
                n153 = Index Array(array=w247, index=1) -> (element=w248:cluster{string[]})
                n154 = call <vilib>:"NT Read String.vi"("name"=w250) -> ("value"=w249:string)  [unwired: 8 in, 2 out]
                n155 = Unbundle(w248) -> (w245:string[])
                n156 = Match First String(2:w245, 3:w249) -> (0:w244:i32)  [unwired: 1 out]
                n157 = property on="Test Ring" class="Ring (strict)"("Value"=w244, "Strings []"=w245) -> ()  [unwired: 2 in, 2 out]
                n158 = property on="Test Ring" class="Ring (strict)"("Visible"=TRUE) -> ()  [unwired: 2 in, 2 out]
                n159 = property on="Test Slider" class="Slide (strict)"("Visible"=FALSE) -> ()  [unwired: 2 in, 2 out]
              }
              frame "Exposure  **" {
                n160 = Index Array(array=w256, index=2) -> (element=w257:cluster{string[]})
                n161 = call <vilib>:"NT Read String.vi"("name"=w259) -> ("value"=w258:string)  [unwired: 8 in, 2 out]
                n162 = Unbundle(w257) -> (w253:string[])
                n163 = Match First String(2:w253, 3:w258) -> (0:w254:i32)  [unwired: 1 out]
                n164 = property on="Test Ring" class="Ring (strict)"("Value"=w254, "Strings []"=w253) -> ()  [unwired: 2 in, 2 out]
                n165 = property on="Test Ring" class="Ring (strict)"("Visible"=TRUE) -> ()  [unwired: 2 in, 2 out]
                n166 = property on="Test Slider" class="Slide (strict)"("Visible"=FALSE) -> ()  [unwired: 2 in, 2 out]
              }
              frame "Exposure Priority  **" {
                n167 = Index Array(array=w265, index=3) -> (element=w266:cluster{string[]})
                n168 = call <vilib>:"NT Read String.vi"("name"=w268) -> ("value"=w267:string)  [unwired: 8 in, 2 out]
                n169 = Unbundle(w266) -> (w262:string[])
                n170 = Match First String(2:w262, 3:w267) -> (0:w263:i32)  [unwired: 1 out]
                n171 = property on="Test Ring" class="Ring (strict)"("Value"=w263, "Strings []"=w262) -> ()  [unwired: 2 in, 2 out]
                n172 = property on="Test Ring" class="Ring (strict)"("Visible"=TRUE) -> ()  [unwired: 2 in, 2 out]
                n173 = property on="Test Slider" class="Slide (strict)"("Visible"=FALSE) -> ()  [unwired: 2 in, 2 out]
              }
              frame "Color Enable  **" {
                n174 = Index Array(array=w274, index=4) -> (element=w275:cluster{string[]})
                n175 = call <vilib>:"NT Read String.vi"("name"=w277) -> ("value"=w276:string)  [unwired: 8 in, 2 out]
                n176 = Unbundle(w275) -> (w271:string[])
                n177 = Match First String(2:w271, 3:w276) -> (0:w272:i32)  [unwired: 1 out]
                n178 = property on="Test Ring" class="Ring (strict)"("Value"=w272, "Strings []"=w271) -> ()  [unwired: 2 in, 2 out]
                n179 = property on="Test Ring" class="Ring (strict)"("Visible"=TRUE) -> ()  [unwired: 2 in, 2 out]
                n180 = property on="Test Slider" class="Slide (strict)"("Visible"=FALSE) -> ()  [unwired: 2 in, 2 out]
              }
              frame Default {
                n181 = property on="Test Ring" class="Ring (strict)"("Visible"=FALSE) -> ()  [unwired: 2 in, 2 out]
                n182 = property on="Test Slider" class="Slide (strict)"("Visible"=FALSE) -> ()  [unwired: 2 in, 2 out]
              }
              frame "Brightness  **", "Color Level  **", "Compression  **", "FPS  **", "Sharpness  **" {
                n183 = call <vilib>:"NT Read Number.vi"("name"=w283) -> ("value"=w282:dbl)  [unwired: 8 in, 2 out]
                n184 = local write "Test Slider"(w282) -> ()
                n185 = property on="Test Ring" class="Ring (strict)"("Visible"=FALSE) -> ()  [unwired: 2 in, 2 out]
                n186 = property on="Test Slider" class="Slide (strict)"("Visible"=TRUE, "Scale.Maximum"=100.0 ("Scale.Range:Maximum")) -> ()  [unwired: 2 in, 2 out]
              }
            }
          }
        }
        n187 = property on="Progress" class="Clust (strict)"("Visible"=FALSE) -> ()  [unwired: 2 in, 2 out]
      }
      event "Test Name": Mouse Enter {
        # "Populate the ring with the list of tests"
        n188 = event-data() -> ()  [unwired: 1 in, 1 out]
        n189 = call <vilib>:"NT Read String Array.vi"("name"="TestMode/TestList" ("Name")) -> ("value"=w290:string[])  [unwired: 8 in, 2 out]
        n190 = Build Array (concatenate)("Select the test to run...", w290) -> (w289:string[])
        n191 = property on="Test Name" class="Ring (strict)"("Strings []"=w289) -> ()  [unwired: 2 in, 2 out]
      }
      event "Test Name": Value Change {
        w291 = FALSE ("Visible")
        # "Tell the robot the test name to run"
        n192 = event-data() -> ("NewVal"=w295:u16)  [unwired: 1 in]
        n193 = property on="Test Name" class="Ring (strict)"() -> ("Strings []"=w296:string[])  [unwired: 2 in, 2 out]
        n194 = local write "Progress"(T6 {"Test Progress"=0, "Test Progress Text"=""} ("Progress")) -> ()
        n195 = Index Array(array=w296, index=w295) -> (element=w294:string)
        n196 = call <vilib>:"NT Write String.vi"("value"=w294, "name"="TestMode/TestName" ("Name")) -> ()  [unwired: 9 in, 1 out]
        n197 = property on="Progress" class="Clust (strict)"("Visible"=TRUE) -> ()  [unwired: 2 in, 2 out]
        n198 = property on="Motor" class="Clust (strict)"("Visible"=w291) -> ()  [unwired: 2 in, 2 out]
        n199 = property on="Test Slider" class="Slide (strict)"("Visible"=w291) -> ()  [unwired: 2 in, 2 out]
        n200 = property on="On/Off" class="Bool (strict)"("Visible"=w291) -> ()  [unwired: 2 in, 2 out]
        n201 = property on="Rev/Fwd" class="Clust (strict)"("Visible"=w291) -> ()  [unwired: 2 in, 2 out]
        n202 = property on="Test Ring" class="Ring (strict)"("Visible"=w291) -> ()  [unwired: 2 in, 2 out]
      }
      event "Select Auto": Mouse Enter {
        # "Populate the combo box with the list of autonomous options"
        n203 = event-data() -> ()  [unwired: 1 in, 1 out]
        n204 = call <vilib>:"NT Read String Array.vi"("name"="Auto List" ("Name")) -> ("value"=w298:string[])  [unwired: 8 in, 2 out]
        n205 = property on="Select Auto" class="CmbBox"("Strings[]"=w298) -> ()  [unwired: 2 in, 2 out]
      }
      event "Select Auto": Value Change {
        # "User modified the Auto Selection. Write to NT variable so robot knows."
        n206 = event-data() -> ("NewVal"=w300:string)  [unwired: 1 in]
        n207 = call <vilib>:"NT Write String.vi"("value"=w300, "name"="Auto Selector" ("Name")) -> ()  [unwired: 9 in, 1 out]
      }
      event "CheckList": Double Click {
        # "Shift clears all"
        # "Update symbols on the listbox"
        n208 = event-data() -> ("PlatMods.Shift"=w302:bool, "Row"=w304:i32)  [unwired: 1 in]
        n209 = case shown="True" w302 {
          tunnel: w304 -> [w308 _]
          tunnel: 1 -> [w307 _]
          frame False {
            n210 = property on="CheckList" class="LstBox (strict)"() -> ("Item Symbols"=w306:i32[])  [unwired: 2 in, 2 out]
            n211 = Replace Array Subset(array=w306, new element=w307, index=w308) -> (w305:i32[])
            n212 = property on="CheckList" class="LstBox (strict)"("Item Symbols"=w305) -> ()  [unwired: 2 in, 2 out]
          }
          frame True {
            w309 = 0 ("Top Row")
            n213 = property on="CheckList" class="LstBox (strict)"() -> ("Number of Rows"=w311:u32)  [unwired: 2 in, 2 out]
            n214 = Initialize Array(0, w311) -> (w310:i32[])
            n215 = property on="CheckList" class="LstBox (strict)"("Top Row"=w309, "Value"=w309, "Item Symbols"=w310) -> ()  [unwired: 2 in, 2 out]
          }
        }
      }
      event "CheckList": Key Down {
        # "Update symbols on the listbox\nLeft and right keys check and uncheck"
        n216 = event-data() -> ("VKey"=w314:T22)  [unwired: 1 in]
        n217 = case shown="\"Left\", \"Right\"" w314 {
          selector: w314 -> [w319 _]
          tunnel: eventvkey."Left" ("VKey") -> [w317 _]
          frame "Left", "Right" {
            n218 = Equal?(x=w317, y=w319) -> (x = y?=w318:bool)
            n219 = Select(t=0, s=w318, f=1) -> (s? t:f=w320:i32)
            n220 = property on="CheckList" class="LstBox (strict)"() -> ("Item Symbols"=w323:i32[])  [unwired: 2 in, 2 out]
            n221 = Replace Array Subset(array=w323, new element=w320, index="CheckList") -> (w322:i32[])
            n222 = property on="CheckList" class="LstBox (strict)"("Item Symbols"=w322) -> ()  [unwired: 2 in, 2 out]
          }
          frame Default {
          }
        }
      }
      event "Motor.Enable": Value Change {
        # "When the test mode otor enable helper is set, update that\ntree row item's value"
        n223 = event-data() -> ("NewVal"=w328:bool)  [unwired: 1 in]
        n224 = Unbundle("Motor") -> ("Value"=w327:dbl)  [unwired: 1 out]
        n225 = Select(t=w327, s=w328, f=0.0) -> (s? t:f=w325:dbl)
        n226 = call <vilib>:"NT Write Number.vi"("value"=w325, "name"=w324) -> ()  [unwired: 9 in, 1 out]
      }
      event "Test Slider": Value Change {
        # "When the test mode slider helper is set, update that\ntree row item's value"
        n227 = event-data() -> ("NewVal"=w330:dbl)  [unwired: 1 in]
        n228 = call <vilib>:"NT Write Number.vi"("value"=w330, "name"=w331) -> ()  [unwired: 9 in, 1 out]
      }
      event "On/Off": Value Change {
        # "When the test mode on/off helper value is set, update that\ntree row item's value"
        n229 = event-data() -> ("NewVal"=w334:bool)  [unwired: 1 in]
        n230 = Boolean To (0,1)(Boolean=w334) -> (0, 1=w333:i16)
        n231 = call <vilib>:"NT Write Number.vi"("value"=w333, "name"=w332) -> ()  [unwired: 9 in, 1 out]
      }
      event "Rev/Fwd": Value Change {
        # "When the test mode helper value for relays is set, update that\ntree row item's value"
        n232 = event-data() -> ("NewVal.Forward"=w341:bool, "NewVal.Reverse"=w340:bool)  [unwired: 1 in]
        n233 = Boolean To (0,1)(Boolean=w341) -> (0, 1=w337:i16)
        n234 = Boolean To (0,1)(Boolean=w340) -> (0, 1=w339:i16)
        n235 = Negate(x=w339) -> (-x=w338:i16)
        n236 = Add(x=w337, y=w338) -> (x+y=w336:i16)
        n237 = call <vilib>:"NT Write Number.vi"("value"=w336, "name"=w335) -> ()  [unwired: 9 in, 1 out]
      }
      event "Test Ring": Value Change {
        # "When a test mode helper value is selected from the ring,\nset the tree item's variable to the string value"
        n238 = event-data() -> ("NewVal"=w344:u16)  [unwired: 1 in]
        n239 = property on="Test Ring" class="Ring (strict)"() -> ("Strings []"=w345:string[])  [unwired: 2 in, 2 out]
        n240 = Index Array(array=w345, index=w344) -> (element=w343:string)
        n241 = call <vilib>:"NT Write String.vi"("value"=w343, "name"=w342) -> ()  [unwired: 9 in, 1 out]
      }
      event "Rec Mode": Value Change {
        # "Update globals for recording mode and path to read log from.\nClear when logging and let NetworkTables set path for vision to\nuse."
        n242 = event-data() -> ("NewVal"=w354:enum32{"Stop", "Record", "Playback"})  [unwired: 1 in]
        n243 = global write "WPI_DashboardLogging Global.vi" "Logging Filename"(path "") -> ()
        n244 = global write "WPI_DashboardLogging Global.vi" "Recording"(w354) -> ()
        n245 = case shown="\"Playback\"" w354 {
          tunnel: w353 -> [_ w356 w364]
          tunnel: [_ _ w363] -> w351
          tunnel: [_ _ w362] -> _
          tunnel: w349 -> [_ _ w360]
          tunnel: cluster{i32, i32} {-250, 170} -> [_ _ w359]
          tunnel: [_ _ T23 {"Image Size"=TRUE, "Image Type"=TRUE, "Pixel Value"=TRUE, "ROI Information"=TRUE, "Zoom Factor"=FALSE} ("Image Information Shown:All Elements")] -> w346
          tunnel: [_ _ TRUE ("Zoom Factor")] -> w347
          frame Default {
          }
          frame "Stop", "Record" {
            # "Place Window too"
            n246 = invoke class="VI" method="FP.Close"(reference=w356) -> (reference out=w355:refnum<vi>)  [unwired: 2 in, 2 out]
            n247 = invoke class="VI" method="Abort VI"(reference=w355) -> ()  [unwired: 2 in, 3 out]
          }
          frame "Playback" {
            n248 = call "Open Playback Panel.vi"("Offset"=w359, "DB VI Ref"=w360, "Playback in"=w364) -> ("Playback out"=w361:refnum<vi>)  [unwired: 8 in]
            n249 = register-events(w361) -> (reference out=w363:refnum<event-registration>, error out=w362:errorcluster)  [unwired: 2 in]
          }
        }
        n250 = property on="Camera Image Right" class="ImageControl"("Image Information Shown"=w346, "Image Information Visible"=w347) -> ()  [unwired: 2 in, 2 out]
        n251 = property on="Camera Image" class="ImageControl"("Image Information Shown"=w346, "Image Information Visible"=w347) -> ()  [unwired: 2 in, 2 out]
        n252 = call <vilib>:"WPI_DashboardNT Log FieldName Cache.vi"("Operation"=enum16{"Lookup/Add", "Index", "Clear"}."Clear") -> ()  [unwired: 8 in, 3 out]
      }
      event Panel Close {
        w365 = enum32{"Stop", "Record", "Playback"}."Stop" ("Rec Mode")
        # "Playback window has been closed, abort"
        n253 = event-data() -> ()  [unwired: 1 in, 4 out]
        n254 = local write "Rec Mode"(w365) -> ()
        n255 = global write "WPI_DashboardLogging Global.vi" "Recording"(w365) -> ()
      }
      event Panel Close {
        # "Abort playback window and ourself"
        n256 = event-data() -> ()  [unwired: 1 in, 4 out]
        n257 = invoke class="VI" method="FP.Close"(reference=w368) -> (reference out=w367:refnum<vi>)  [unwired: 2 in, 2 out]
        n258 = invoke class="VI" method="Abort VI"(reference=w367) -> (error out=w366:errorcluster)  [unwired: 2 in, 2 out]
        n259 = invoke class="VI" method="Abort VI"(error in=w366) -> ()  [unwired: 2 in, 3 out]
      }
      event "Tree": Double Click {
        n260 = event-data() -> ("PlatMods"=w374:T25, "Tag"=w371:string)  [unwired: 1 in]
        n261 = Unbundle(w374) -> ("Shift"=w373:bool)  [unwired: 4 out]
        n262 = String Subset(string=w371, length (rest)=1 ("length (rest)")) -> (substring=w370:string)  [unwired: 1 in]
        n263 = Not(x=w373) -> (.not. x?=w372:bool)
        n264 = case shown="\"/\"" w370 {
          tunnel: w371 -> [_ w376]
          tunnel: w372 -> [_ w375]
          frame Default {
          }
          frame "/" {
            n265 = call <vilib>:"NT Update Persistence.vi"("Persistence"=w375, "Name"=w376) -> ()  [unwired: 9 in, 1 out]
          }
        }
      }
    }
  }
  n266 = while {
    tunnel: w54 -> [w378]
    i -> [w381]
    stop <- FALSE stop-if-true
    n267 = Wait (ms)(milliseconds to wait=u32 100) -> ()  [unwired: 1 out]
    n268 = case shown="\"Playback\"" "Rec Mode" {
      tunnel: w381 -> [_ _ w396]
      tunnel: [u32 2829099 ("Base Color") u32 11141120 ("Target Color") w385] -> w377
      frame "Stop", Default {
        # "Reset the color, extra updates don't cost much"
      }
      frame "Record" {
      }
      frame "Playback" {
        # "Playback"
        n269 = Quotient & Remainder(x=w396, y=u32 50 ("milliseconds to wait")) -> (x-y*floor(x/y)=w392:u32)  [unwired: 1 out]
        n270 = Divide(x=w392, y=u32 50 ("milliseconds to wait")) -> (x/y=w389:dbl)
        n271 = Multiply(x=6.283185307179586, y=w389) -> (x*y=w394:dbl)
        n272 = Sine(x=w394) -> (sin(x)=w393:dbl)
        n273 = Absolute Value(x=w393) -> (abs(x)=w386:dbl)
        n274 = call "Interpolate RGB Color.vi"("Proportion"=w386, "Target Color"=u32 30976, "Base Color"=u32 2829099) -> ("Result Color"=w385:u32)  [unwired: 8 in]
      }
    }
    n275 = property class="Pane"(reference=w378, "PaneColor"=w377) -> ()  [unwired: 1 in, 2 out]
  }
  n276 = local write "Dashboard Tab"(T2."Drive" ("Dashboard Tab")) -> ()
  n277 = property on="On/Off" class="Bool (strict)"("Visible"=w26) -> ()  [unwired: 2 in, 2 out]
  n278 = property on="Motor" class="Clust (strict)"("Visible"=w26) -> ()  [unwired: 2 in, 2 out]
  n279 = property on="Progress" class="Clust (strict)"("Visible"=w26) -> ()  [unwired: 2 in, 2 out]
  n280 = property on="Test Ring" class="Ring (strict)"("Visible"=w26) -> ()  [unwired: 2 in, 2 out]
  n281 = property on="Rev/Fwd" class="Clust (strict)"("Visible"=w26) -> ()  [unwired: 2 in, 2 out]
  n282 = while {
    tunnel: u16 1741 ("timeout ms (25000)") -> [w398]
    stop <- FALSE stop-if-true
    n283 = TCP Create Listener(10:w398) -> (0:w397:errorcluster, 3:w399:refnum<k5>)  [unwired: 4 in, 1 out]
    n284 = case shown="No Error" w397 {
      selector: w397 -> [w401 _]
      tunnel: w399 -> [w402 _]
      frame No Error {
        n285 = while {
          tunnel: w402 -> [w405]
          tunnel: w401 -> [w404]
          stop <- FALSE stop-if-true
          n286 = TCP Wait On Listener(8:w404, 11:w405) -> (0:w406:errorcluster, 4:w407:refnum<k5>)  [unwired: 2 in, 3 out]
          n287 = local write "TCP"(w407) -> ()
          n288 = case shown="Error" w406 {
            frame No Error {
            }
            frame Error {
              n289 = Wait (ms)(milliseconds to wait=u32 1000) -> ()  [unwired: 1 out]
            }
          }
        }
      }
      frame Error {
        n290 = Wait (ms)(milliseconds to wait=u32 1000) -> ()  [unwired: 1 out]
      }
    }
  }
  n291 = global write "WPI_DashboardLogging Global.vi" "Recording"(w49) -> ()
  n292 = local write "Rec Mode"(w49) -> ()
  n293 = call <vilib>:"NT Write String.vi"("value"="Select Auto", "name"="Auto Selector" ("Name")) -> ()  [unwired: 9 in, 1 out]
